vi "(SubVI) PSD Cut_YCC.vi"(4 "PSD":dbl[](array[numeric]), 5 "Freq End Cut":dbl, 6 "Freq Strat Cut":dbl, 7 "Frequency (Hz)":dbl[](array[numeric])) -> (0 "PSD Cut":dbl[](array[numeric]), 3 "Freq Cut":dbl[](array[numeric]))   [LabVIEW 2014]
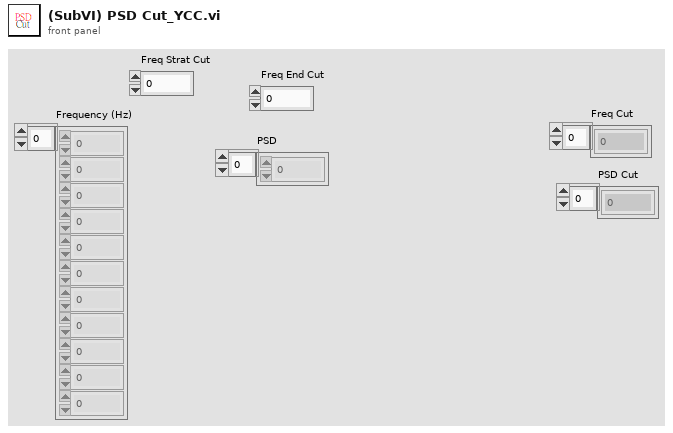
[diagram p1: front panel]
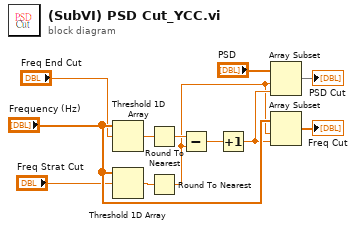
[diagram p0: block diagram]
diagram:
  n1 = Threshold 1D Array(2:"Freq End Cut", 3:"Frequency (Hz)") -> (0:w8:dbl)  [unwired: 1 in]
  n2 = Threshold 1D Array(2:"Freq Strat Cut", 3:"Frequency (Hz)") -> (0:w11:dbl)  [unwired: 1 in]
  n3 = Round To Nearest(number=w8) -> (nearest integer value=w7:dbl)
  n4 = Round To Nearest(number=w11) -> (nearest integer value=w1:dbl)
  n5 = Subtract(x=w7, y=w1) -> (x-y=w6:dbl)
  n6 = Increment(x=w6) -> (x+1=w5:dbl)
  n7 = Array Subset(array="PSD", index=w1, length=w5) -> (→"PSD Cut":dbl[])
  n8 = Array Subset(array="Frequency (Hz)", index=w1, length=w5) -> (→"Freq Cut":dbl[])
